vi "setUserEvents.vi"(10 "UserEvents":refnum<class "UserEvents.lvclass">, 11 "M1M3SAL in":refnum<class "M1M3SAL.lvclass">) -> (3 "M1M3SAL out":refnum<class "M1M3SAL.lvclass">)   [LabVIEW 2016, in "M1M3SupportCommunicator.lvlib" / "M1M3SAL.lvclass"]
uses:
  M1M3SAL.lvclass
  UserEvents/UserEvents.lvclass
  M1M3SAL.lvclass/M1M3SAL.ctl
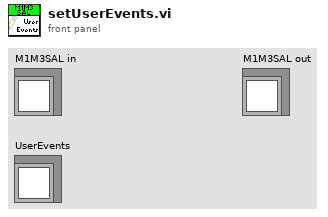
[diagram p1: front panel]
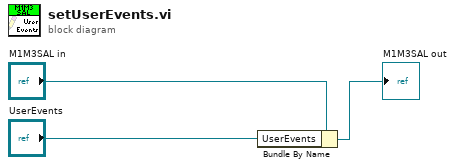
[diagram p0: block diagram]
diagram:
  n1 = Bundle By Name(cluster="M1M3SAL in", "UserEvents"="UserEvents") -> (→"M1M3SAL out":refnum<class "M1M3SAL.lvclass">)
